vi "input-validation.vi"(8 "error constant":errorcluster, 9 "Ki-xy":sgl=0.005, 11 "z-axis-params":T1={"TOL"=0.3, "ramp_rate"=0.0, "z_u_max"=5.0, "setpoint"=0.0, "Ki"=0.0, "Z_error_threshold"=0.0, "Z_settled_samples_threshold "=0, "z_UP"=1.5, "zup_N"=5000} {"Z_error_threshold" format="%#_13g"; "ramp_rate" format="%#_13g"; "TOL" format="%#_13g"}) -> (0 "error out":errorcluster)   [LabVIEW 2017]
uses:
  z-axis-params.ctl
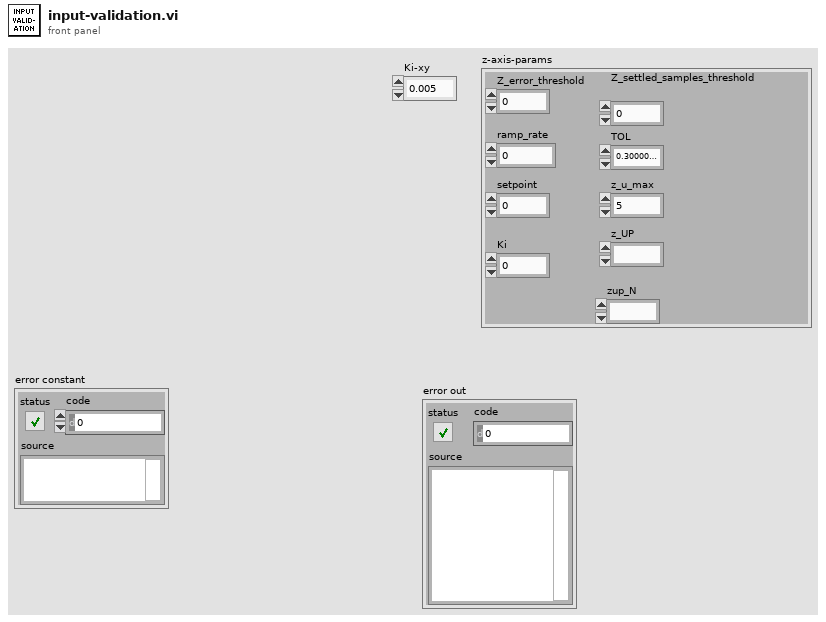
[diagram p1: front panel]
types:
  T1 = typedef "z-axis-params.ctl" = cluster{"TOL":sgl, "ramp_rate":sgl, "z_u_max":sgl, "setpoint":sgl, "Ki":sgl, "Z_error_threshold":sgl, "Z_settled_samples_threshold ":i16, "z_UP":fxp<+/-,16,5>, "zup_N":i16}
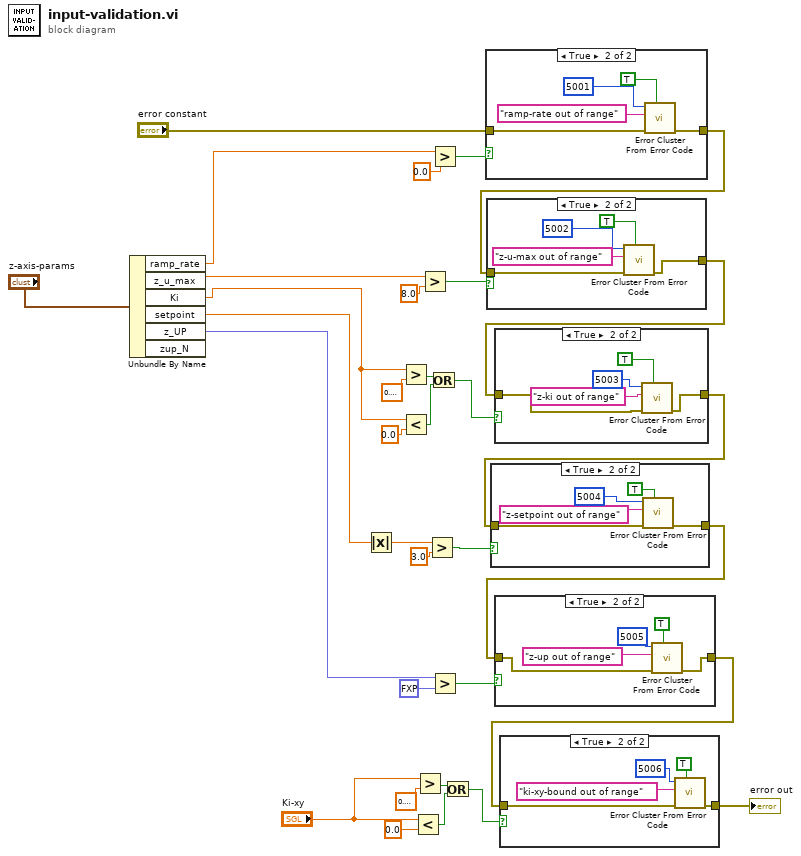
[diagram p0: block diagram]
diagram:
  n1 = Unbundle By Name("z-axis-params") -> ("ramp_rate"=w27:sgl, "z_u_max"=w25:sgl, "Ki"=w5:sgl, "setpoint"=w4:sgl, "z_UP"=w3:fxp<+/-,16,5>)  [unwired: 1 out]
  n2 = Absolute Value(x=w4) -> (abs(x)=w31:sgl)
  n3 = Greater?(x=w5, y=sgl 0.1) -> (0:w14:bool)
  n4 = Less?(x=w5, y=sgl 0.0) -> (x < y?=w15:bool)
  n5 = Less?(x="Ki-xy", y=sgl 0.0) -> (x < y?=w9:bool)
  n6 = Greater?(x="Ki-xy", y=sgl 0.1) -> (0:w10:bool)
  n7 = Greater?(x=w25, y=sgl 8.0) -> (0:w12:bool)
  n8 = Greater?(x=w31, y=sgl 3.0) -> (0:w18:bool)
  n9 = Or(x=w14, y=w15) -> (x .or. y?=w13:bool)
  n10 = Greater?(x=w27, y=sgl 0.0) -> (0:w22:bool)
  n11 = Greater?(x=w3, y=fxp<+/-,16,5> 5.0) -> (0:w16:bool)
  n12 = Or(x=w10, y=w9) -> (x .or. y?=w8:bool)
  n13 = case shown="True" w22 {
    tunnel: "error constant" -> [w34 w39]
    tunnel: [w34 w35] -> w21
    frame False {
    }
    frame True {
      n14 = call <vilib>:"Error Cluster From Error Code.vi"("show call chain? (False)"=TRUE, "error in (no error)"=w39, "error message (\"\")"="ramp-rate out of range", "error code (0)"=5001) -> ("error out"=w35:errorcluster)  [unwired: 5 in]
    }
  }
  n15 = case shown="True" w12 {
    tunnel: w21 -> [w40 w43]
    tunnel: [w40 w44] -> w20
    frame False {
    }
    frame True {
      n16 = call <vilib>:"Error Cluster From Error Code.vi"("show call chain? (False)"=TRUE, "error in (no error)"=w43, "error message (\"\")"="z-u-max out of range", "error code (0)"=5002) -> ("error out"=w44:errorcluster)  [unwired: 5 in]
    }
  }
  n17 = case shown="True" w13 {
    tunnel: w20 -> [w46 w47]
    tunnel: [w46 w48] -> w19
    frame False {
    }
    frame True {
      n18 = call <vilib>:"Error Cluster From Error Code.vi"("show call chain? (False)"=TRUE, "error in (no error)"=w47, "error message (\"\")"="z-ki out of range", "error code (0)"=5003) -> ("error out"=w48:errorcluster)  [unwired: 5 in]
    }
  }
  n19 = case shown="True" w18 {
    tunnel: w19 -> [w52 w55]
    tunnel: [w52 w56] -> w17
    frame False {
    }
    frame True {
      n20 = call <vilib>:"Error Cluster From Error Code.vi"("show call chain? (False)"=TRUE, "error in (no error)"=w55, "error message (\"\")"="z-setpoint out of range", "error code (0)"=5004) -> ("error out"=w56:errorcluster)  [unwired: 5 in]
    }
  }
  n21 = case shown="True" w16 {
    tunnel: w17 -> [w58 w59]
    tunnel: [w58 w63] -> w1
    frame False {
    }
    frame True {
      n22 = call <vilib>:"Error Cluster From Error Code.vi"("show call chain? (False)"=TRUE, "error in (no error)"=w59, "error message (\"\")"="z-up out of range", "error code (0)"=5005) -> ("error out"=w63:errorcluster)  [unwired: 5 in]
    }
  }
  n23 = case shown="True" w8 {
    tunnel: [w64 w66] -> w2
    tunnel: w1 -> [w64 w67]
    frame False {
    }
    frame True {
      n24 = call <vilib>:"Error Cluster From Error Code.vi"("show call chain? (False)"=TRUE, "error in (no error)"=w67, "error message (\"\")"="ki-xy-bound out of range", "error code (0)"=5006) -> ("error out"=w66:errorcluster)  [unwired: 5 in]
    }
  }
  "error out" <- w2
